vi "Autodetect SLSC Switch Module Configuration.vi"(8 "error in":errorcluster, 10 "slsc module":refnum<k21>, 11 "slsc switch custom device in":T1 format="%.0x") -> (0 "error out":errorcluster, 3 "slsc switch custom device out":T1 format="%.0x")   [LabVIEW 2017, in "SLSC Switch Scripting.lvlib"]
uses:
  SLSC Switch Scripting.lvlib
  <vilib>/NI Veristand/Custom Device API/Custom Device Item Ref.ctl
  <vilib>/NI Veristand/Custom Device API/Custom Device API.lvlib
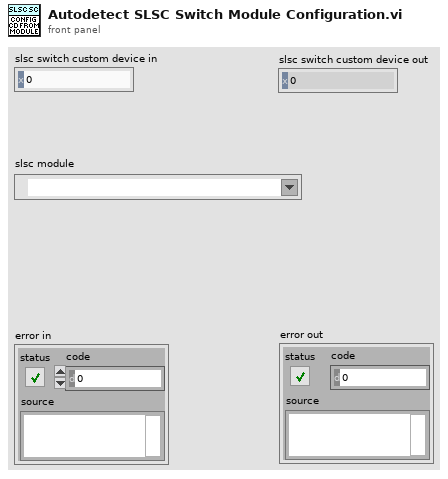
[diagram p1: front panel]
types:
  T1 = typedef "Custom Device API.lvlib/Custom Device Item Ref.ctl" = u64
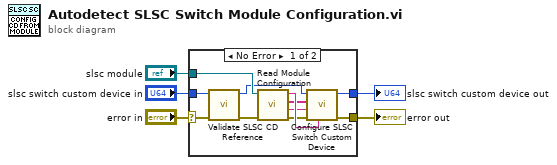
[diagram p0: block diagram]
diagram:
  n1 = case shown="No Error" "error in" {
    selector: "error in" -> [w9 w17]
    tunnel: "slsc switch custom device in" -> [w8 w18]
    tunnel: [w16 w17] -> w1
    tunnel: "slsc module" -> [w13 _]
    tunnel: [w15 w18] -> w2
    frame No Error {
      n2 = call "Validate SLSC CD Reference.vi"("error in (no error)"=w9, "SLSC Switch Custom Device Ref in"=w8) -> ("error out"=w6:errorcluster, "SLSC Switch Custom Device Ref out"=w7:T1)  [unwired: 8 in]
      n3 = call "Read Module Configuration.vi"("error in (no error)"=w6, "SLSC Device"=w13) -> ("error out"=w12:errorcluster, "switches json"=w10:string, "topologies"=w11:string[], "product name"=w14:string)  [unwired: 5 in, 1 out]
      n4 = call "Configure SLSC Switch Custom Device.vi"("product name"=w14, "error in (no error)"=w12, "switches json"=w10, "topologies"=w11, "SLSC Switch Custom Device Ref in"=w7) -> ("error out"=w16:errorcluster, "SLSC Switch Custom Device Ref out"=w15:T1)  [unwired: 5 in]
    }
    frame Error {
    }
  }
  "error out" <- w1
  "slsc switch custom device out" <- w2
